vi "InitCurveResults.vi"(2 "Measurements In":T1, 3 "Curves By Measurement In":T4, 4 "Active Measurement":refnum<k24>, 5 "Curve Index":i32) -> (0 "Curves By Measurement Out":T4, 1 "Measurements Out":T1)   [LabVIEW 2025]
uses:
  E:/PSCode/PalmSens_SDK/labview/PalmSens/Libraries/PalmSens.Core.Simplified.LabVIEW.dll
  Libraries/PalmSens.Core.Simplified.LabVIEW.dll
  CurvesByMeasurement.ctl
  MeasurementInfo.ctl
  LiveCurveResult.ctl
  CurveInfo.ctl
  MeasurementsResult.ctl
  MeasurementResults.ctl
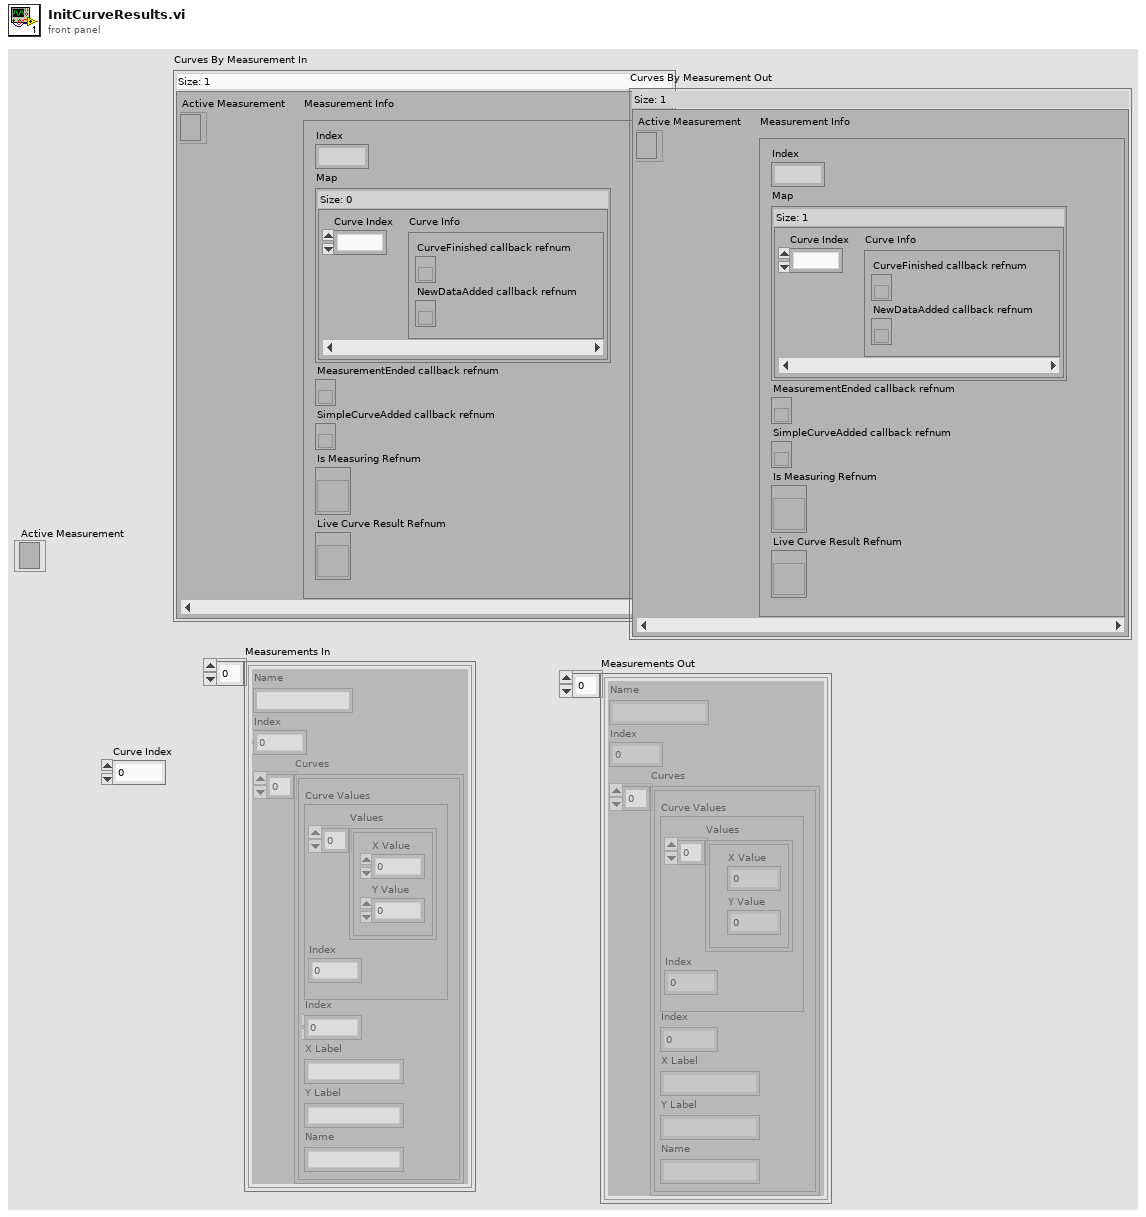
[diagram p1: front panel]
types:
  T1 = typedef "MeasurementsResult.ctl" = cluster{"Name":string, "Curves":T2, "Index":i32}[]
  T2 = typedef "MeasurementResults.ctl" = T3[]
  T3 = typedef "LiveCurveResult.ctl" = cluster{"X Label":string, "Y Label":string, "Name":string, "Index":i16, "Curve Values":cluster{"Values":cluster{"X Value":dbl, "Y Value":dbl}[], "Index":i16}}
  T4 = typedef "CurvesByMeasurement.ctl" = map{refnum<k24>, T5}
  T5 = typedef "MeasurementInfo.ctl" = cluster{"Index":i32, "Is Measuring Refnum":refnum<vi>, "MeasurementEnded callback refnum":refnum<k27>, "SimpleCurveAdded callback refnum":refnum<k27>, "Live Curve Result Refnum":refnum<vi>, "Map":map{i32, T6}}
  T6 = typedef "CurveInfo.ctl" = cluster{"NewDataAdded callback refnum":refnum<k27>, "CurveFinished callback refnum":refnum<k27>}
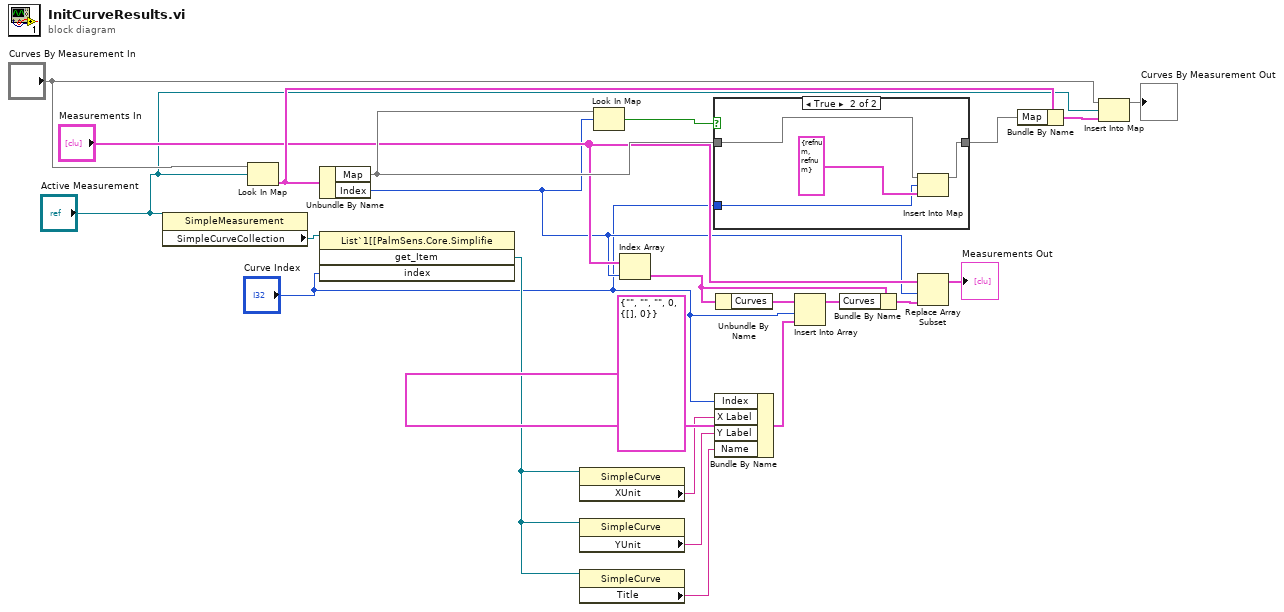
[diagram p0: block diagram]
diagram:
  n1 = property class="SimpleMeasurement"(reference="Active Measurement") -> ("SimpleCurveCollection"=w2:refnum<k24>)  [unwired: 1 in, 2 out]
  n2 = Look In Map(map="Curves By Measurement In", key="Active Measurement") -> (value=w23:T5)  [unwired: 1 in, 1 out]
  n3 = Unbundle By Name(w23) -> ("Map"=w15:map{i32, T6}, "Index"=w5:i32)
  n4 = invoke class="List`1[[PalmSens.Core.Simplifie" method="get_Item"(reference=w2, "index"="Curve Index") -> ("get_Item"=w4:refnum<k24>)  [unwired: 2 in, 3 out]
  n5 = property class="SimpleCurve"(reference=w4) -> ("XUnit"=w6:string)  [unwired: 1 in, 2 out]
  n6 = property class="SimpleCurve"(reference=w4) -> ("YUnit"=w7:string)  [unwired: 1 in, 2 out]
  n7 = property class="SimpleCurve"(reference=w4) -> ("Title"=w8:string)  [unwired: 1 in, 2 out]
  n8 = Look In Map(map=w15, key=w5) -> (key not found?=w16:bool)  [unwired: 1 in, 1 out]
  n9 = Index Array(array="Measurements In", index=w5) -> (element=w19:cluster{"Name":string, "Curves":T2, "Index":i32})
  n10 = case shown="True" w16 {
    tunnel: w15 -> [w24 w28]
    tunnel: [w24 w27] -> w14
    tunnel: "Curve Index" -> [_ w25]
    frame False {
    }
    frame True {
      n11 = Insert Into Map(map in=w28, key=w25, value=T6 {"NewDataAdded callback refnum"=refnum, "CurveFinished callback refnum"=refnum}) -> (map out=w27:map{i32, T6})  [unwired: 2 out]
    }
  }
  n12 = Bundle By Name(cluster=T3 {"X Label"="", "Y Label"="", "Name"="", "Index"=0, "Curve Values"={"Values"=[], "Index"=0}} ("Cluster"), "Index"="Curve Index", "X Label"=w6, "Y Label"=w7, "Name"=w8) -> (w21:T3)
  n13 = Unbundle By Name(w19) -> ("Curves"=w20:T2)
  n14 = Insert Into Array(array=w20, index="Curve Index", new element=w21) -> (w18:T2)
  n15 = Bundle By Name(cluster=w19, "Curves"=w18) -> (w17:cluster{"Name":string, "Curves":T2, "Index":i32})
  n16 = Replace Array Subset(array="Measurements In", new element=w17, index=w5) -> (→"Measurements Out":T1)
  n17 = Bundle By Name(cluster=w23, "Map"=w14) -> (w22:T5)
  n18 = Insert Into Map(map in="Curves By Measurement In", key="Active Measurement", value=w22) -> (map out=→"Curves By Measurement Out":T4)  [unwired: 2 out]
